vi "Read Groups.vi"(8 "error in (no error)":errorcluster, 11 "ParseSVG in":refnum<class "ParseSVG.lvclass">) -> (0 "error out":errorcluster, 2 "Groups":T1(array[cluster]), 3 "ParseSVG out":refnum<class "ParseSVG.lvclass">)   [LabVIEW 2019, in "ParseSVG.lvclass"]
uses:
  ParseSVG.lvclass
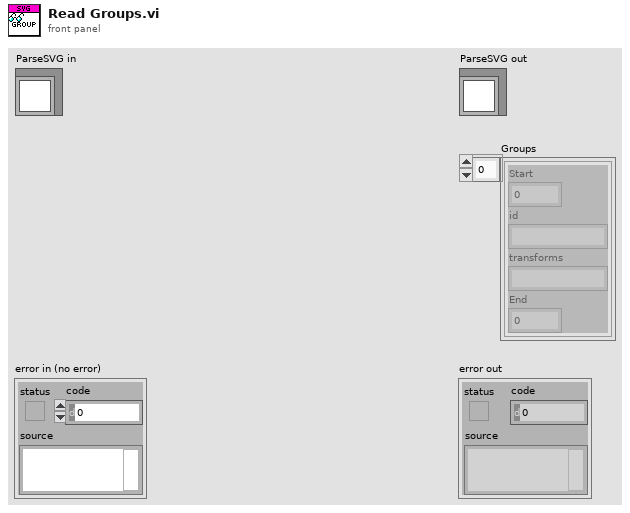
[diagram p1: front panel]
types:
  T1 = cluster{"Start":i32, "id":string, "transforms":string, "End":i32}[]
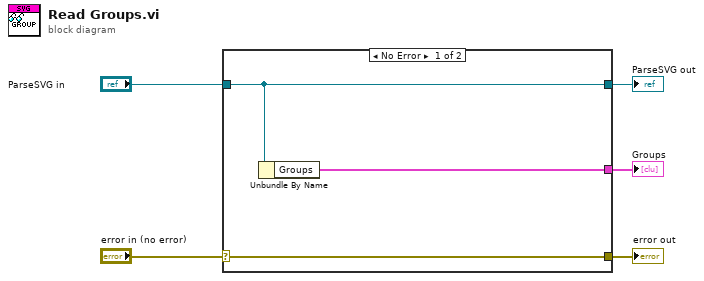
[diagram p0: block diagram]
diagram:
  n1 = case shown="No Error" "error in (no error)" {
    selector: "error in (no error)" -> [w8 w9]
    tunnel: [w8 w9] -> w4
    tunnel: [w7 w10] -> w2
    tunnel: "ParseSVG in" -> [w7 w10]
    tunnel: [w6 _] -> w1
    frame No Error {
      n2 = Unbundle By Name(w7) -> ("Groups"=w6:T1)
    }
    frame Error {
    }
  }
  "error out" <- w4
  "ParseSVG out" <- w2
  "Groups" <- w1
